vi "USB_Comm.vi"() -> ()   [LabVIEW 2016]
uses:
  VIs/uPythonX/uPythonX.xctl
panel:
  in  "Other":T1(xcontrol)={"VISA Refnum in"="ASRL44::INSTR", "All Code"="eval('1+1')\n\nexec('fred = 2')\n\nexec(\n'''\nfred = 2\nfred = fred + 2\nprint(fred)\n'''\n)"}
  in  "USB_VCP":T1(xcontrol)={"VISA Refnum in"="ASRL44::INSTR", "All Code"="'''\nhttp://docs.micropython.org/en/v1.9.3/pyboard/library/pyb.USB_VCP.html\n'''\n\nimport pyb,utime\n\nfred = pyb.USB_VCP()\n\ntest = ['hi\\n','bye\\n','ok\\n']\n\nwhile True:\n     if fred.any():\n          value = fred.read(fred.any())\n          try:\n               fred.write(test[int(value)])\n          except:\n               pass\n     utime.sleep_ms(100)"}
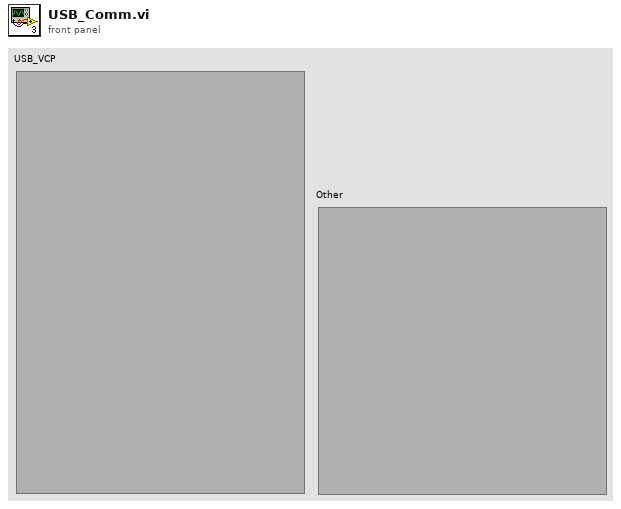
[diagram p1: front panel]
types:
  T1 = cluster{"VISA Refnum in":refnum<visa-resource-name>, "All Code":string}
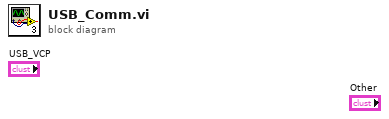
[diagram p0: block diagram]
diagram:
